vi "Lipid Quantification.vi"() -> ()   [LabVIEW 2013]
uses:
  <vilib>/vision/NI_Vision_Development_Module.lvlib
panel:
  in  "Tab Control":enum32{"ROI", "FOV"}(tab)
  out "ROI":T1(graph)
  out "FOV":T1(graph)
  in  "Search offset (pixels)":i16=80
  in  "Template offset (pixels)":i16=40
  in  "Interval (sec)":dbl=5.0
  in  "Minimum match score":dbl
  out "# of analyzed images:":dbl=11.0
  out "Total # of images:":i32=1329
  out "Stabilized":T2(plugin-control)
  out "Reference Image":T2(plugin-control)
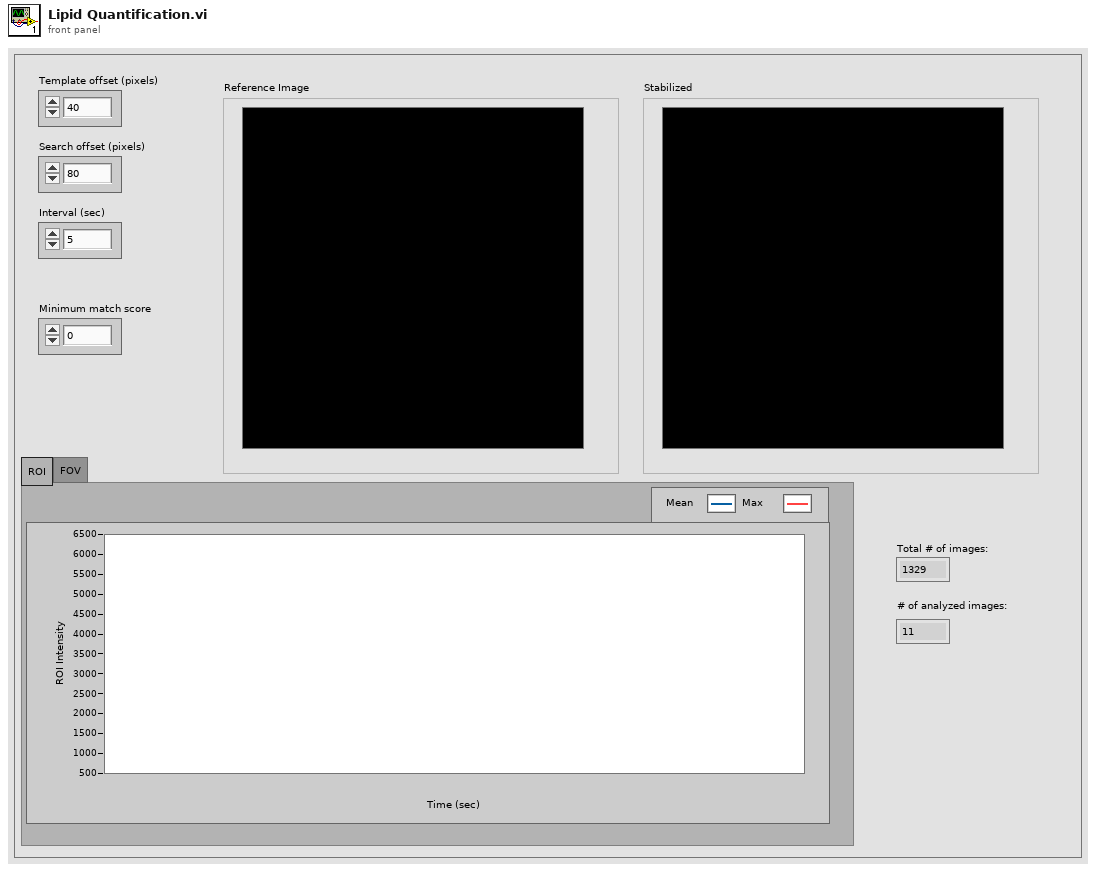
[diagram p1: front panel]
types:
  T1 = cluster{"Mean Intensity":sgl, "Maximum Intensity":sgl}
  T2 = typedef "IMAQ Image.ctl" = refnum<image>
  T3 = cluster{"Mean Intensity":sgl, "Maximum Intensity":sgl}[]
  T4 = typedef "Image Type" = u32
  T5 = typedef "IMAQ Rectangle" = cluster{"Left":i32, "Top":i32, "Right":i32, "Bottom":i32, "Rotation":dbl}
  T6 = cluster{"Left":i32, "Top":i32, "Right":i32, "Bottom":i32}
  T7 = typedef "ROI Descriptor" = cluster{"Global Rectangle":i32[], "Contours":cluster{"ID":enum32{"External", "Internal"}, "Type":u32, "Coordinates":i32[]}[]}
  T8 = cluster{"Position":cluster{"x":sgl, "y":sgl}, "Angle":sgl, "Scale":sgl, "Score":sgl, "Bounding Box":cluster{"x":sgl, "y":sgl}[]}[]
  T9 = cluster{"Mean Intensity":sgl, "Standard  Deviation":sgl, "Minimum Intensity":sgl, "Maximum Intensity":sgl}
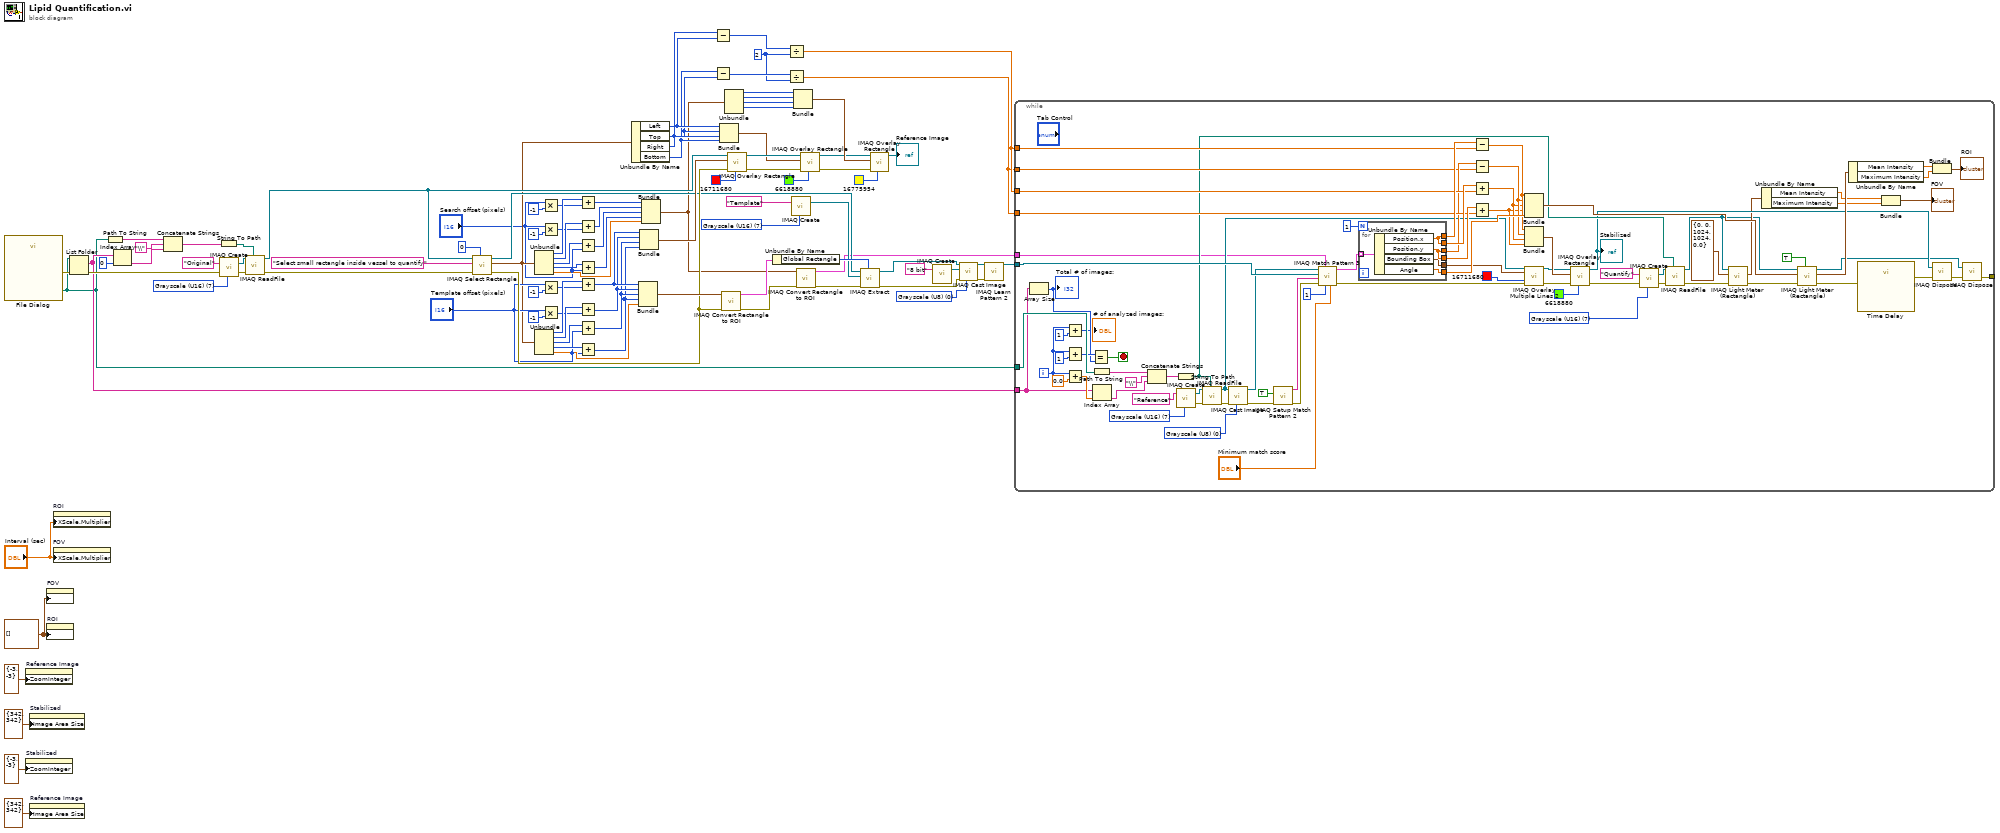
[diagram p0: block diagram]
diagram:
  w1 = T3 [] ("History Data")
  w35 = T4 0 items=["Grayscale (U8)", "Grayscale (I16)", "Grayscale (SGL)", "Complex (CSG)", "RGB (U32)", "HSL (U32)", "RGB (U64)", "Grayscale (U16)"] ("Image Type")
  w40 = T4 7 items=["Grayscale (U8)", "Grayscale (I16)", "Grayscale (SGL)", "Complex (CSG)", "RGB (U32)", "HSL (U32)", "RGB (U64)", "Grayscale (U16)"] ("Image Type")
  w41 = T4 7 items=["Grayscale (U8)", "Grayscale (I16)", "Grayscale (SGL)", "Complex (CSG)", "RGB (U32)", "HSL (U32)", "RGB (U64)", "Grayscale (U16)"] ("Image Type")
  w47 = 2 ("y")
  n1 = call "File Dialog"() -> ("selected path"=w56:path, "error out"=w96:errorcluster)  [unwired: 12 in, 2 out]
  n2 = property on="Reference Image" class="ImageControl"("ZoomInteger"=cluster{"X":i32, "Y":i32} {"X"=-3, "Y"=-3} ("ZoomInteger:All Elements")) -> ()  [unwired: 2 in, 2 out]
  n3 = property on="Stabilized" class="ImageControl"("ZoomInteger"=cluster{"X":i32, "Y":i32} {"X"=-3, "Y"=-3} ("ZoomInteger:All Elements")) -> ()  [unwired: 2 in, 2 out]
  n4 = property on="Stabilized" class="ImageControl"("Image Area Size"=cluster{"Width":u32, "Height":u32} {"Width"=342, "Height"=342} ("Image Area:Size:All Elements")) -> ()  [unwired: 2 in, 2 out]
  n5 = property on="Reference Image" class="ImageControl"("Image Area Size"=cluster{"Width":u32, "Height":u32} {"Width"=342, "Height"=342} ("Image Area:Size:All Elements")) -> ()  [unwired: 2 in, 2 out]
  n6 = property on="FOV" class="WFChart (strict)"("History Data"=w1) -> ()  [unwired: 2 in, 2 out]
  n7 = property on="ROI" class="WFChart (strict)"("History Data"=w1) -> ()  [unwired: 2 in, 2 out]
  n8 = property on="ROI" class="WFChart (strict)"("XScale.Multiplier"="Interval (sec)") -> ()  [unwired: 2 in, 2 out]
  n9 = property on="FOV" class="WFChart (strict)"("XScale.Multiplier"="Interval (sec)") -> ()  [unwired: 2 in, 2 out]
  n10 = List Folder(path=w56, error in=w96) -> (filenames=w57:string[], error out=w97:errorcluster)  [unwired: 2 in, 2 out]
  n11 = Path To String(path=w56) -> (string=w93:string)
  n12 = Index Array(array=w57, index=0) -> (element=w90:string)
  n13 = Concatenate Strings(w93, "\\" ("string"), w90) -> (w92:string)
  n14 = String To Path(string=w92) -> (path=w91:path)
  n15 = call "IMAQ Create"("Image Name"="Original", "Image Type"=w41, "error in (no error)"=w97) -> ("New Image"=w88:T2, "error out"=w94:errorcluster)  [unwired: 2 in]
  n16 = call "IMAQ ReadFile"("File Path"=w91, "error in (no error)"=w94, "Image"=w88) -> ("error out"=w42:errorcluster, "Image Out"=w43:T2)  [unwired: 4 in, 3 out]
  n17 = call "IMAQ Select Rectangle"("Window Number (0...15)"=0, "error in (no error)"=w42, "Prompt"="Select small rectangle inside vessel to quantify", "Image In"=w43) -> ("error out"=w61:errorcluster, "Rectangle"=w17:T5, "Image Out (duplicate)"=w38:T2)  [unwired: 4 in, 1 out]
  n18 = Unbundle(w17) -> ("Left"=w30:i32, "Top"=w29:i32, "Right"=w28:i32, "Bottom"=w27:i32, "Rotation"=w18:dbl)
  n19 = Unbundle(w17) -> ("Left"=w84:i32, "Top"=w83:i32, "Right"=w82:i32, "Bottom"=w81:i32, "Rotation"=w65:dbl)
  n20 = Multiply(x="Search offset (pixels)", y=-1) -> (x*y=w23:i32)
  n21 = Multiply(x="Search offset (pixels)", y=-1) -> (x*y=w26:i32)
  n22 = Multiply(x="Template offset (pixels)", y=-1) -> (x*y=w75:i32)
  n23 = Multiply(x="Template offset (pixels)", y=-1) -> (x*y=w78:i32)
  n24 = Add(x=w30, y=w23) -> (x+y=w22:i32)
  n25 = Add(x=w29, y=w26) -> (x+y=w21:i32)
  n26 = Add(x=w28, y="Search offset (pixels)") -> (x+y=w20:i32)
  n27 = Add(x=w27, y="Search offset (pixels)") -> (x+y=w19:i32)
  n28 = Add(x=w84, y=w75) -> (x+y=w69:i32)
  n29 = Add(x=w83, y=w78) -> (x+y=w68:i32)
  n30 = Add(x=w82, y="Template offset (pixels)") -> (x+y=w67:i32)
  n31 = Add(x=w81, y="Template offset (pixels)") -> (x+y=w66:i32)
  n32 = Unbundle By Name(w17) -> ("Left"=w52:i32, "Top"=w50:i32, "Right"=w53:i32, "Bottom"=w51:i32)
  n33 = Bundle(w69, w68, w67, w66, "Rotation"=w65) -> (w64:cluster{i32, i32, i32, i32, "Rotation":dbl})  [unwired: 1 in]
  n34 = Bundle(w69, w68, w67, w66) -> (w70:cluster{i32, i32, i32, i32})  [unwired: 1 in]
  n35 = Bundle(w22, w21, w20, w19, "Rotation"=w18) -> (w10:cluster{i32, i32, i32, i32, "Rotation":dbl})  [unwired: 1 in]
  n36 = Subtract(x=w53, y=w52) -> (x-y=w49:i32)
  n37 = Subtract(x=w51, y=w50) -> (x-y=w48:i32)
  n38 = Bundle("Left"=w52, "Top"=w50, "Right"=w53, "Bottom"=w51) -> (w72:T6)  [unwired: 1 in]
  n39 = call "IMAQ Convert Rectangle to ROI"("error in (no error)"=w61, "Rectangle"=w64) -> ("error out"=w15:errorcluster, "ROI Descriptor"=w63:T7)  [unwired: 7 in]
  n40 = Unbundle(w10) -> (w9:i32, w8:i32, w7:i32, w6:i32)  [unwired: 1 out]
  n41 = call "IMAQ Overlay Rectangle"("Color"=u32 16711680, "error in (no error)"=w61, "Rectangle"=w70, "Image"=w43) -> ("error out"=w73:errorcluster, "Image Out"=w74:T2)  [unwired: 6 in]
  n42 = Unbundle By Name(w63) -> ("Global Rectangle"=w62:i32[])
  n43 = Divide(x=w49, y=w47) -> (x/y=w46:dbl)
  n44 = Divide(x=w48, y=w47) -> (x/y=w45:dbl)
  n45 = call "IMAQ Create"("Image Name"="Template", "Image Type"=w40) -> ("New Image"=w59:T2)  [unwired: 3 in, 1 out]
  n46 = Bundle(w9, w8, w7, w6) -> (w5:cluster{i32, i32, i32, i32})  [unwired: 1 in]
  n47 = call "IMAQ Convert Rectangle to ROI"("error in (no error)"=w15, "Rectangle"=w10) -> ("error out"=w14:errorcluster, "ROI Descriptor"=w13:T7)  [unwired: 7 in]
  n48 = call "IMAQ Overlay Rectangle"("Color"=u32 6618880, "error in (no error)"=w73, "Rectangle"=w72, "Image"=w74) -> ("error out"=w12:errorcluster, "Image Out"=w4:T2)  [unwired: 6 in]
  n49 = call "IMAQ Extract"("Optional Rectangle"=w62, "error in (no error)"=w14, "Image Dst"=w59, "Image Src"=w38) -> ("error out"=w31:errorcluster, "Image Dst Out"=w34:T2)  [unwired: 6 in]
  n50 = call "IMAQ Overlay Rectangle"("Color"=u32 16775954, "error in (no error)"=w12, "Rectangle"=w5, "Image"=w4) -> ("Image Out"=→"Reference Image":T2)  [unwired: 6 in, 1 out]
  n51 = call "IMAQ Create"("Image Name"="8 bit") -> ("New Image"=w36:T2)  [unwired: 4 in, 1 out]
  n52 = call "IMAQ Cast Image"("Image Type"=w35, "error in (no error)"=w31, "Image Dst"=w36, "Image Src"=w34) -> ("error out"=w32:errorcluster, "Image Dst Out"=w33:T2)  [unwired: 6 in]
  n53 = call "IMAQ Learn Pattern 2"("error in (no error)"=w32, "Image"=w33) -> ("Template Image Out"=w58:T2)  [unwired: 8 in, 1 out]
  n54 = while {
    tunnel: w58 -> [w176]
    tunnel: w57 -> [w163]
    tunnel: w56 -> [w170]
    tunnel: w46 -> [w156]
    tunnel: w46 -> [w154]
    tunnel: w45 -> [w152]
    tunnel: w45 -> [w150]
    tunnel: [w118] -> _
    tunnel: w13 -> [w110]
    i -> [w130]
    stop <- w162 stop-if-true
    w109 = T4 7 items=["Grayscale (U8)", "Grayscale (I16)", "Grayscale (SGL)", "Complex (CSG)", "RGB (U32)", "HSL (U32)", "RGB (U64)", "Grayscale (U16)"] ("Image Type")
    w113 = T4 0 items=["Grayscale (U8)", "Grayscale (I16)", "Grayscale (SGL)", "Complex (CSG)", "RGB (U32)", "HSL (U32)", "RGB (U64)", "Grayscale (U16)"] ("Image Type")
    w114 = T4 7 items=["Grayscale (U8)", "Grayscale (I16)", "Grayscale (SGL)", "Complex (CSG)", "RGB (U32)", "HSL (U32)", "RGB (U64)", "Grayscale (U16)"] ("Image Type")
    n55 = Array Size(array=w163) -> (size(s)=w159:i32)
    "Total # of images:" <- w159
    n56 = Add(x=w130, y=1) -> (x+y=→"# of analyzed images:":i32)
    n57 = Add(x=w130, y=1) -> (x+y=w160:i32)
    n58 = Add(x=w130, y=0.0) -> (x+y=w166:dbl)
    n59 = Equal?(x=w160, y=w159) -> (x = y?=w162:bool)
    n60 = Path To String(path=w170) -> (string=w165:string)
    n61 = Index Array(array=w163, index=w166) -> (element=w164:string)
    n62 = Concatenate Strings(w165, "\\" ("string"), w164) -> (w173:string)
    n63 = String To Path(string=w173) -> (path=w123:path)
    n64 = call "IMAQ Create"("Image Name"="Reference", "Image Type"=w114) -> ("New Image"=w171:T2, "error out"=w174:errorcluster)  [unwired: 3 in]
    n65 = call "IMAQ ReadFile"("File Path"=w123, "error in (no error)"=w174, "Image"=w171) -> ("error out"=w116:errorcluster, "Image Out"=w111:T2)  [unwired: 4 in, 3 out]
    n66 = call "IMAQ Cast Image"("Image Type"=w113, "error in (no error)"=w116, "Image Src"=w111) -> ("error out"=w115:errorcluster, "Image Dst Out"=w112:T2)  [unwired: 7 in]
    n67 = call "IMAQ Setup Match Pattern 2"("error in (no error)"=w115, "Subpixel Accuracy"=TRUE) -> ("error out"=w134:errorcluster, "Match Pattern Setup Data"=w132:string)  [unwired: 8 in]
    n68 = call "IMAQ Match Pattern 3"("Minimum Match Score"="Minimum match score", "Number of Matches Requested"=1, "ROI Descriptor"=w110, "error in (no error)"=w134, "Match Pattern Setup Data"=w132, "Template Image"=w176, "Image"=w112) -> ("error out"=w146:errorcluster, "Matches"=w168:T8)  [unwired: 2 in, 1 out]
    n69 = for {
      N: 1 -> [_]
      tunnel: w168 -> [w181] mode=indexing
      tunnel: [w180] -> w157
      tunnel: [w180] -> w155
      tunnel: [w179] -> w153
      tunnel: [w179] -> w151
      tunnel: [w178] -> w149
      tunnel: [w177] -> w147
      n70 = Unbundle By Name(w181) -> ("Position.x"=w180:sgl, "Position.y"=w179:sgl, "Bounding Box"=w177:cluster{"x":sgl, "y":sgl}[], "Angle"=w178:sgl)
    }
    n71 = Subtract(x=w157, y=w156) -> (x-y=w145:dbl)
    n72 = Subtract(x=w151, y=w150) -> (x-y=w144:dbl)
    n73 = Add(x=w155, y=w154) -> (x+y=w143:dbl)
    n74 = Add(x=w153, y=w152) -> (x+y=w142:dbl)
    n75 = Bundle(w145, w144, w143, w142, "Angle"=w149) -> (w148:cluster{dbl, dbl, dbl, dbl, "Angle":sgl})  [unwired: 1 in]
    n76 = Bundle(w145, w144, w143, w142) -> (w141:cluster{dbl, dbl, dbl, dbl})  [unwired: 1 in]
    n77 = call "IMAQ Overlay Multiple Lines 2"("Image"=w111, "Line End Points"=w147, "Color"=u32 16711680, "error in (no error)"=w146) -> ("Image Out"=w140:T2, "error out"=w139:errorcluster)  [unwired: 10 in]
    n78 = call "IMAQ Overlay Rectangle"("Color"=u32 6618880, "error in (no error)"=w139, "Rectangle"=w141, "Image"=w140) -> ("error out"=w122:errorcluster, "Image Out"=w121:T2)  [unwired: 6 in]
    "Stabilized" <- w121
    n79 = call "IMAQ Create"("Image Name"="Quantify", "Image Type"=w109, "error in (no error)"=w122) -> ("New Image"=w125:T2, "error out"=w126:errorcluster)  [unwired: 2 in]
    n80 = call "IMAQ ReadFile"("File Path"=w123, "error in (no error)"=w126, "Image"=w125) -> ("error out"=w106:errorcluster, "Image Out"=w107:T2)  [unwired: 4 in, 3 out]
    n81 = call "IMAQ Light Meter (Rectangle)"("error in (no error)"=w106, "Rectangle"=T5 {"Left"=0, "Top"=0, "Right"=1024, "Bottom"=1024, "Rotation"=0.0}, "Image"=w107) -> ("error out"=w105:errorcluster, "Gray Level Intensities"=w108:T9)  [unwired: 4 in, 3 out]
    n82 = Unbundle By Name(w108) -> ("Mean Intensity"=w103:sgl, "Maximum Intensity"=w102:sgl)
    n83 = call "IMAQ Light Meter (Rectangle)"("Show Search Area"=TRUE, "error in (no error)"=w105, "Rectangle"=w148, "Image"=w107) -> ("error out"=w136:errorcluster, "Gray Level Intensities"=w137:T9, "Image Out"=w119:T2)  [unwired: 3 in, 2 out]
    n84 = Unbundle By Name(w137) -> ("Mean Intensity"=w100:sgl, "Maximum Intensity"=w99:sgl)
    n85 = call "Time Delay"("error in (no error)"=w136) -> ("error out"=w135:errorcluster)  [unwired: 10 in]
    n86 = Bundle("Mean Intensity"=w103, "Maximum Intensity"=w102) -> (→"FOV":T1)  [unwired: 1 in]
    n87 = Bundle("Mean Intensity"=w100, "Maximum Intensity"=w99) -> (→"ROI":T1)  [unwired: 1 in]
    n88 = call "IMAQ Dispose"("Image"=w121, "error in (no error)"=w135) -> ("error out"=w120:errorcluster)  [unwired: 4 in]
    n89 = call "IMAQ Dispose"("Image"=w119, "error in (no error)"=w120) -> ("error out"=w118:errorcluster)  [unwired: 4 in]
  }
